vi "TreePopup.vi"(10 "TreeView Value":string, 11 "Menu in":refnum<k9>) -> (2 "ItemTagToName":map{string, string}(c390))   [LabVIEW 2021, in "ScriptManager.lvlib"]
uses:
  ScriptManager.lvlib
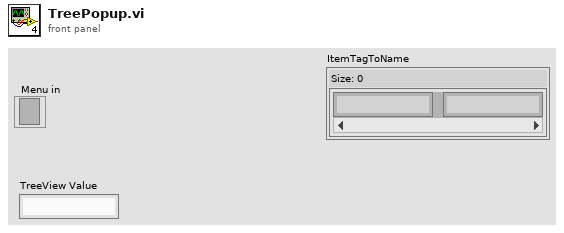
[diagram p1: front panel]
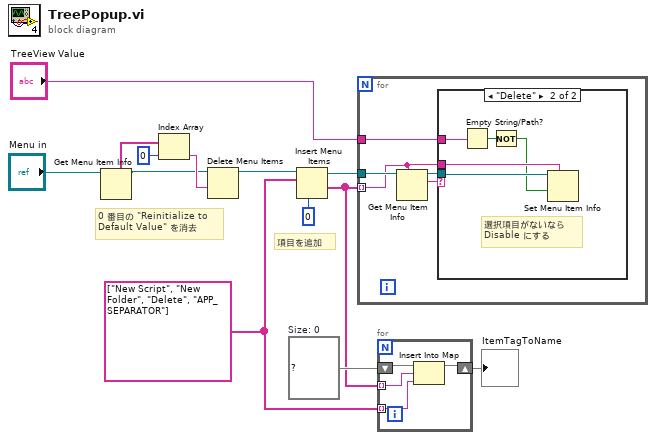
[diagram p0: block diagram]
diagram:
  w4 = map{string, string} {}  # Size: 0
  w2 = string[] ["New Script", "New Folder", "Delete", "APP_SEPARATOR"]
  # "項目を追加"
  # "0 番目の \"Reinitialize to \nDefault Value\" を消去"
  n1 = Get Menu Item Info(11:"Menu in") -> (3:w5:refnum<k9>, 5:w6:string[])  [unwired: 2 in, 5 out]
  n2 = Index Array(array=w6, index=0) -> (element=w8:string)
  n3 = Delete Menu Items(7:w8, 9:w5) -> (3:w10:refnum<k9>)  [unwired: 2 in, 1 out]
  n4 = Insert Menu Items(4:0, 8:w2, 9:w10) -> (1:w3:string[], 3:w12:refnum<k9>)  [unwired: 3 in, 1 out]
  n5 = for {
    tunnel: w3 -> [w14] mode=indexing
    tunnel: w12 -> [w18]
    tunnel: "TreeView Value" -> [w16]
    n6 = Get Menu Item Info(7:w14, 11:w18) -> (2:w17:string, 3:w15:refnum<k9>)  [unwired: 1 in, 5 out]
    n7 = case shown="\"Delete\"" w17 {
      tunnel: w16 -> [_ w23]
      tunnel: w15 -> [_ w22]
      tunnel: w14 -> [_ w21]
      frame Default {
      }
      frame "Delete" {
        # "選択項目がないなら\nDisable にする"
        n8 = Empty String/Path?(string/path=w23) -> (empty?=w20:bool)
        n9 = Not(x=w20) -> (.not. x?=w19:bool)
        n10 = Set Menu Item Info(7:w21, 9:w19, 11:w22) -> ()  [unwired: 4 in, 2 out]
      }
    }
  }
  n11 = for {
    tunnel: w3 -> [w26] mode=indexing
    shift-right: [w24] -> w1
    shift-left: w4 -> [w27]
    tunnel: w2 -> [w25] mode=indexing
    n12 = Insert Into Map(map in=w27, key=w26, value=w25) -> (map out=w24:map{string, string})  [unwired: 2 out]
  }
  "ItemTagToName" <- w1
